vi "Read Size.vi"(9 "Decoration in":refnum<class "Decoration.lvclass">) -> (3 "Decoration out":refnum<class "Decoration.lvclass">, 4 "Size":T1)   [LabVIEW 2014, in "Decoration.lvclass"]
uses:
  Decoration.lvclass
  <vilib>/Utility/miscctls.llb/LVBoundsTypeDef.ctl
  Decoration.lvclass/Decoration.ctl
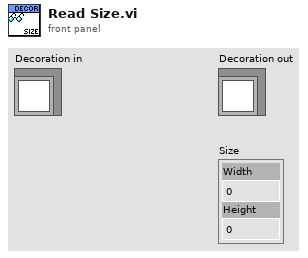
[diagram p1: front panel]
types:
  T1 = typedef "LVBoundsTypeDef.ctl" = cluster{"Width":u32, "Height":u32}
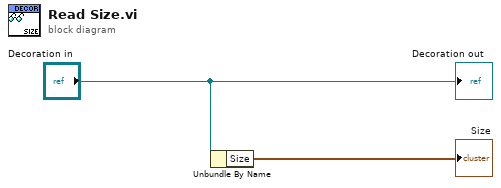
[diagram p0: block diagram]
diagram:
  n1 = Unbundle By Name("Decoration in") -> ("Size"=→"Size":T1)
  "Decoration out" <- "Decoration in"
